vi "#199-SyncMessages.vi"   [LabVIEW 2014]
uses:
  user.lib/_NEVSTOP/Communicable State Machine(CSM)/_Support/Priority Queue/Priority Queue.lvclass/Priority Queue.ctl
  user.lib/_NEVSTOP/Communicable State Machine(CSM)/_Support/Process/CSMP-Sync Call.vi
  user.lib/_NEVSTOP/Communicable State Machine(CSM)/Utility/uuid.vi
  user.lib/_NEVSTOP/Communicable State Machine(CSM)/Utility/Trim Both Whitespace.vi
  user.lib/_NEVSTOP/Communicable State Machine(CSM)/_Support/CSMQ/_CSMObj-Message Check.vi
  user.lib/_NEVSTOP/Communicable State Machine(CSM)/_Support/CSMQ/_CSMObj-Enqueue Cross-Module Message.vi
  user.lib/_NEVSTOP/Communicable State Machine(CSM)/_Support/CSMQ/_CSMOFGV Get.vi
  user.lib/_NEVSTOP/Communicable State Machine(CSM)/_Support/Priority Queue/Enqueue Element.vi
  user.lib/_NEVSTOP/Communicable State Machine(CSM)/Utility/Build Error Cluster.vi
  user.lib/_NEVSTOP/Communicable State Machine(CSM)/_Support/CSMQ/_CSMOFGV.vi
  user.lib/_NEVSTOP/Communicable State Machine(CSM)/Communicable State Machine.lvlib
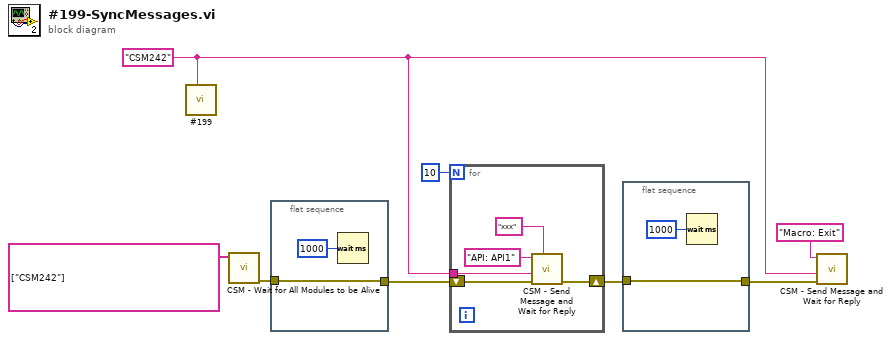
[diagram p0: block diagram]
diagram:
  w2 = "CSM242" ("Name(\"\" to use uuid)")
  n1 = call "#199.vi"("Name(\"\" to use uuid)"=w2) -> ()  [unwired: 11 in]
  n2 = call "CSM - Wait for All Modules to be Alive.vi"("Module Names (in)"=string[] ["CSM242"]) -> ("Error out"=w7:errorcluster)  [unwired: 8 in, 2 out]
  n3 = flat-sequence {
    tunnel: [w9] -> w6
    tunnel: w7 -> [w9]
    frame #0 {
      n4 = Wait (ms)(milliseconds to wait=u32 1000) -> ()  [unwired: 1 out]
    }
  }
  n5 = for {
    N: 10 -> [_]
    tunnel: w2 -> [w12]
    shift-right: [w13] -> w5
    shift-left: w6 -> [w15]
    n6 = call "CSM - Send Message and Wait for Reply.vi"("Current Module(\"\" to generate a ID)"="xxx" ("Current Module(\"\" to generate a ID)"), "Error In (no error)"=w15, "Target Module"=w12, "State"="API: API1") -> ("error out"=w13:errorcluster)  [unwired: 5 in, 2 out]
  }
  n7 = flat-sequence {
    tunnel: [w16] -> w3
    tunnel: w5 -> [w16]
    frame #0 {
      n8 = Wait (ms)(milliseconds to wait=u32 1000) -> ()  [unwired: 1 out]
    }
  }
  n9 = call "CSM - Send Message and Wait for Reply.vi"("Error In (no error)"=w3, "Target Module"=w2, "State"="Macro: Exit") -> ()  [unwired: 6 in, 3 out]
